vi "InitializeExpDepsFilesWithActualDeps.vi"() -> ()   [LabVIEW 2023, in "DepsWatchToolsMenu.lvlib"]
uses:
  DepsWatchToolsMenu.lvlib
  vi.lib/DepsWatch/Typedefs/CICDPathConfigs.ctl
  <userlib>/_OpenG.lib/file/file.llb/File Exists - Scalar__ogtk.vi
  <userlib>/_OpenG.lib/file/file.llb/openg_file.lvlib
  vi.lib/DepsWatch/DepsWatch.lvlib
  <vilib>/Utility/config.llb/NI_LVConfig.lvlib
panel:
  out "ExpectedDeps Files Created":path[](array[path])
  out "error out":errorcluster
  in  "Build Specs Folder Path":path=path "C:/sw-deps-monitor/Source/BuildSpecs"
  in  "error in (no error)":errorcluster
  in  "Source Folder Path":path=path "C:/sw-deps-monitor/Source"
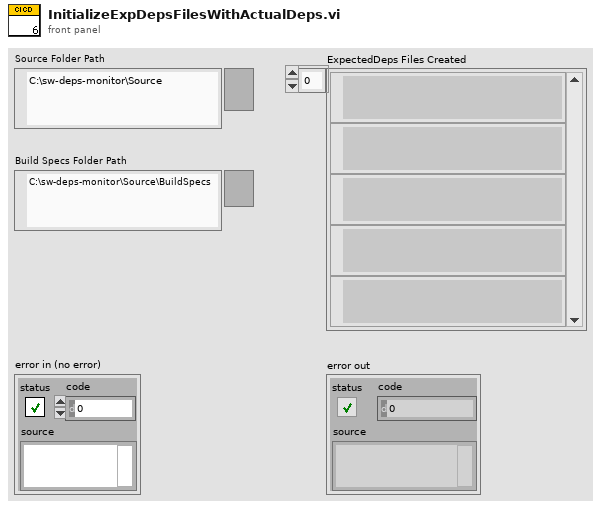
[diagram p1: front panel]
types:
  T1 = typedef "DepsWatch.lvlib/CICDPathConfigs.ctl" = cluster{"GlobalIncludePaths":path[], "GlobalExcludePaths":path[], "BuildSpecsIncludePaths":path[], "ActualDepsIncludePaths":path[], "WorkspacePath":path, "SourceFolderPaths":path[], "ChangedFilesLogpaths":map{string, path}}
  T2 = typedef "NI_LVConfig.lvlib/Config Data RefNum.ctl" = refnum<k1>
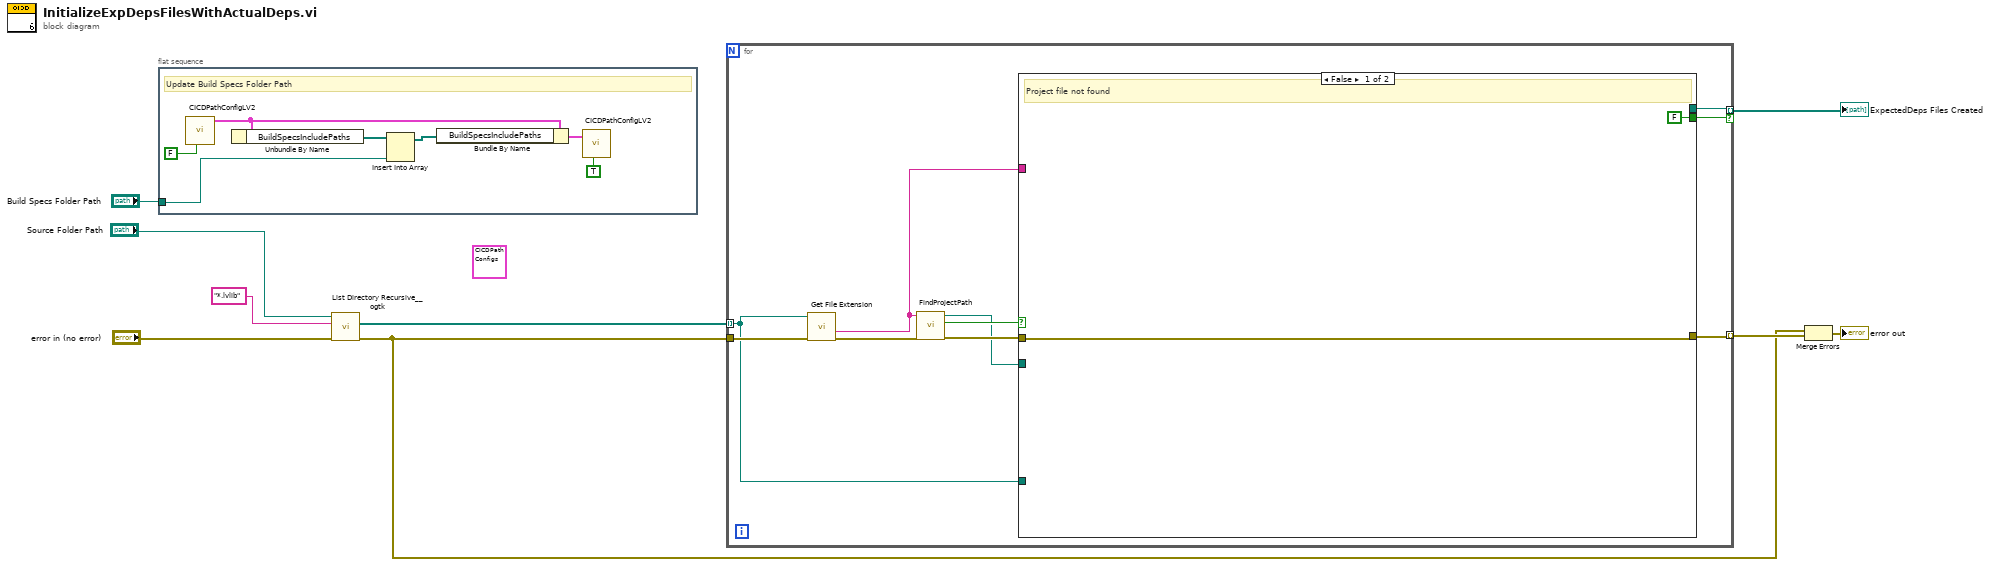
[diagram p0: block diagram]
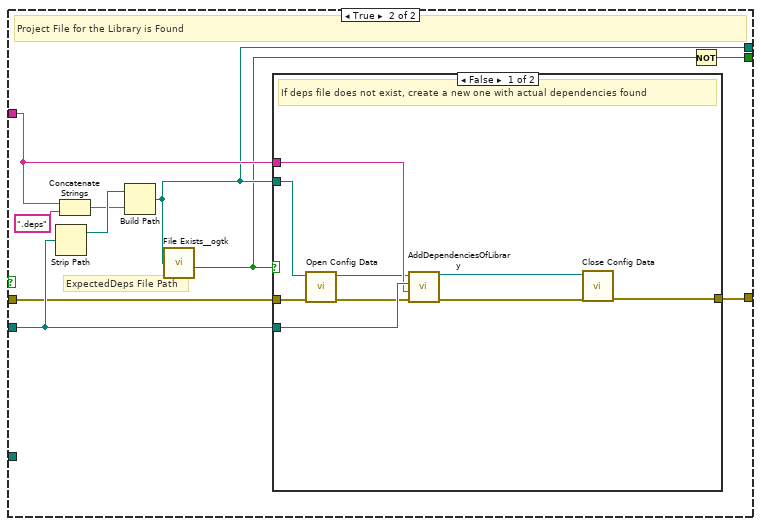
[diagram p2: hidden frame]
diagram:
  (unwired) T1 {"GlobalIncludePaths"=[], "GlobalExcludePaths"=[], "BuildSpecsIncludePaths"=[], "ActualDepsIncludePaths"=[], "WorkspacePath"=path "", "SourceFolderPaths"=[], "ChangedFilesLogpaths"={}} ("CICD Path Config In")
  n1 = flat-sequence {
    tunnel: "Build Specs Folder Path" -> [w13]
    frame #0 {
      # "Update Build Specs Folder Path"
      n2 = call "CICDPathConfigLV2.vi"("Set? (F)"=FALSE) -> ("CICD Path Config Out"=w15:T1)  [unwired: 10 in]
      n3 = Unbundle By Name(w15) -> ("BuildSpecsIncludePaths"=w14:path[])
      n4 = Insert Into Array(array=w14, new element=w13) -> (w12:path[])  [unwired: 1 in]
      n5 = Bundle By Name(cluster=w15, "BuildSpecsIncludePaths"=w12) -> (w11:T1)
      n6 = call "CICDPathConfigLV2.vi"("Set? (F)"=TRUE, "CICD Path Config In"=w11) -> ()  [unwired: 9 in, 1 out]
    }
  }
  n7 = call <userlib>:"List Directory Recursive__ogtk.vi"("error in (no error)"="error in (no error)", "pattern"="*.lvlib", "Path"="Source Folder Path") -> ("error out"=w4:errorcluster, "file paths"=w6:path[])  [unwired: 5 in, 2 out]
  n8 = for {
    tunnel: w4 -> [w26]
    tunnel: w6 -> [w24] mode=indexing
    tunnel: [w25] -> w5 mode=indexing
    tunnel: [w19] -> w2 mode=indexing if=w18
    n9 = call <vilib>:"Get File Extension.vi"("error in (no error)"=w26, "file"=w24) -> ("error out"=w23:errorcluster, "filename without extension"=w17:string)  [unwired: 5 in, 3 out]
    n10 = call "FindProjectPath.vi"("error in (no error)"=w23, "Library Name"=w17) -> ("error out"=w21:errorcluster, "Found?"=w22:bool, "Project Path"=w20:path)  [unwired: 7 in]
    n11 = case shown="False" w22 {
      tunnel: w21 -> [w28 w35]
      tunnel: w24 -> [_ _]
      tunnel: [w28 w32] -> w25
      tunnel: w20 -> [_ w38]
      tunnel: w17 -> [_ w33]
      tunnel: [_ w31] -> w19
      tunnel: [FALSE w29] -> w18
      frame False {
        # "Project file not found"
      }
      frame True {
        # "ExpectedDeps File Path"
        # "Project File for the Library is Found"
        n12 = Strip Path(path=w38) -> (stripped path=w37:path)  [unwired: 1 out]
        n13 = Concatenate Strings(w33, ".deps" ("string")) -> (w36:string)
        n14 = Build Path(base path=w37, name or relative path=w36) -> (appended path=w31:path)
        n15 = call-poly <userlib>:"File Exists__ogtk.vi"("file path"=w31) -> ("exists"=w30:bool)  [unwired: 6 in, 1 out]
        n16 = case shown="False" w30 {
          tunnel: w38 -> [w47 _]
          tunnel: w35 -> [w46 w48]
          tunnel: w31 -> [w45 _]
          tunnel: w33 -> [w43 _]
          tunnel: [w39 w48] -> w32
          frame False {
            # "If deps file does not exist, create a new one with actual dependencies found"
            n17 = call <vilib>:"Open Config Data.vi"("error in (no error)"=w46, "configuration file path"=w45) -> ("error out"=w44:errorcluster, "refnum"=w42:T2)  [unwired: 7 in, 1 out]
            n18 = call "AddDependenciesOfLibrary.vi"("error in (no error)"=w44, "LibraryName"=w43, "Project Path"=w47, "Config Refnum in"=w42) -> ("error out"=w41:errorcluster, "Config Refnum out"=w40:T2)  [unwired: 5 in, 1 out]
            n19 = call <vilib>:"Close Config Data.vi"("error in (no error)"=w41, "refnum"=w40) -> ("error out"=w39:errorcluster)  [unwired: 8 in, 1 out]
          }
          frame True {
          }
        }
        n20 = Not(x=w30) -> (.not. x?=w29:bool)
      }
    }
  }
  "ExpectedDeps Files Created" <- w2
  n21 = Merge Errors(w4, w5) -> (→"error out":errorcluster)
